vi "UiSchematic_b2g1.vi"() -> ()   [LabVIEW 2011]
uses:
  VentilS.ctl
  Pumpe.ctl
  MR.ctl
  Regelventil.ctl
  Output - Cluster b2g1.ctl
  <vilib>/Platform/TimedLoop/XDataNode/timing_clust.ctl
  <vilib>/Platform/TimedLoop/XDataNode/nitl_modes.ctl
  <vilib>/Platform/TimedLoop/XDataNode/wakeup.ctl
  <vilib>/Platform/TimedLoop/XDataNode/XDataNode.xnode
  <vilib>/Platform/TimedLoop/XDataNode/XDNodeRunTimeDep.lvlib
panel:
  out "V-13":T1
  out "V-15":T1
  out "P-9":bool
  out "target connection":bool
  out "TS-6 [°C]":dbl format="%.2g"
  out "HS-2":bool
  in  "Output Var B2G1":refnum<k21>="ni.var.psp://10.27.40.24/variables - b2g1/data - network - b2g1"
  in  "stop":bool
  out "P-4 ERR":bool
  out "P-5 ERR":bool
  out "TS-5 [°C]":dbl format="%.2g"
  out "P-4":T2
  out "DFS-1 [dl]":u64
  out "DFS-1 [l/min]":dbl format="%.2f"
  out "P-4 [%]":u8
  out "P-5 [%]":u8
  out "V-14":T3
  out "V-33":T3
  out "HS-1":bool
  out "pHS-1 [pH]":dbl format="%.2g"
  out "TS-4 [°C]":dbl format="%.2g"
  out "DS-1 [bar]":dbl format="%.2g"
  out "V-13":u8
  out "V-15":u8
  out "P-5":T2
  out "T-2 Max!":bool
  out "T-2 Min!":bool
  out "T-1 Min!":bool
  out "T-1 Max!":bool
  out "V-10":T3
  out "MR Min!":bool
  out "MR Max!":bool
  out "V-34":T3
  out "FS-1 [l]":dbl(slide) scale=10.0..80.0 scale format="%#.2g"
  out "FS-2 [l]":dbl(slide) scale=10.0..80.0 scale format="%#.2g"
  out "FS-3 [l]":T4 scale=0.0..5.0 scale format="%#.1g"
  # "B2G1"
  # "T-3"
  # "T-1"
  # "MR"
  # "T-2"
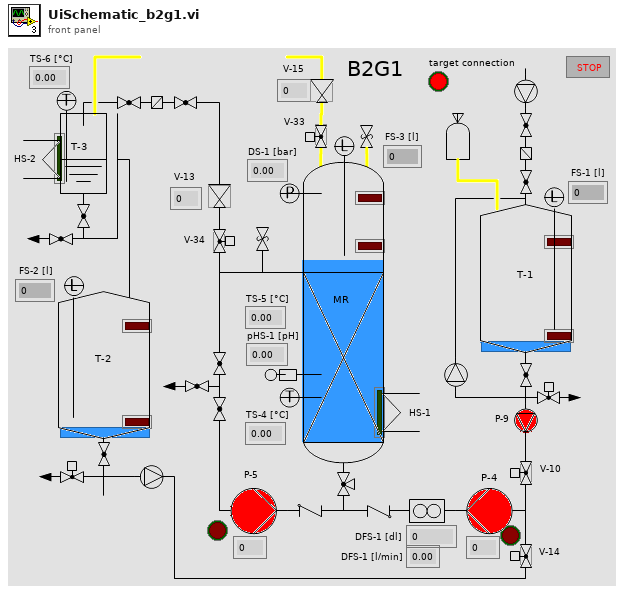
[diagram p1: front panel]
types:
  T1 = typedef "Regelventil.ctl" = bool
  T2 = typedef "Pumpe.ctl" = bool
  T3 = typedef "VentilS.ctl" = bool
  T4 = typedef "MR.ctl" = dbl
  T5 = typedef "Output - Cluster b2g1.ctl" = cluster{"DFS-1 [dl]":u64, "FS-3 [l]":dbl, "DFS-1 [l/min]":dbl, "DS-1 [bar]":dbl, "V-10 ZU":bool, "V-14 ZU":bool, "FS-1 [l]":dbl, "FS-2 [l]":dbl, "TS-4 [°C]":dbl, "HS-1":bool, "V-13 [%]":u8, "V-15 [%]":u8, "P-4 [%]":u8, "P-5 [%]":u8, "Dosierung":bool, "MR Max Füllstand":bool, "MR Min Füllstand":bool, "Dosiermenge [l]":sgl, "V-14 AUF":bool, "V-10 AUF":bool, "T-1 Max Füllstand":bool, "T-1 Min Füllstand":bool, "T-2 Max Füllstand":bool, "T-2 Min Füllstand":bool, "pHS-1 [pH]":dbl, "P-4 RUN":bool, "P-5 RUN ":bool, "V-33 AUF":bool, "V-33 ZU":bool, "V-34 AUF":bool, "V-34 ZU":bool, "P-4 ERR":bool, "P-5 ERR":bool, "TS-5 [°C]":dbl, "TS-6 [°C]":dbl, "P-9 RUN":bool, "HS-2":bool}
  T6 = typedef "XDNodeRunTimeDep.lvlib/timing_clust.ctl" = cluster{"Expected End [f-1]":u64, "Actual End [f-1]":u64, "Finished Late? [f-1]":bool, "Expected End [i-1]":u64, "Actual End [i-1]":u64, "Finished Late? [i-1]":bool, "Expected Start [i]":u64, "Actual Start [i]":u64, "Expected Start [f]":u64, "Actual Start [f]":u64, "Source Name":string, "Structure Name":string, "Period":i64, "Deadline":i64, "Offset":i64, "Start":i64, "Priority":i32, "Timeout":i32, "Mode":T7, "Wakeup Reason":T8, "Error":errorcluster, "Source Type":string, "Secondary Source Type":string, "Global End Time":u64, "Global Start Time":u64, "Frame Duration":u64, "Iteration Duration":u64, "Assigned CPU":i32, "I/O Scan Engine Mode":u32}
  T7 = typedef "XDNodeRunTimeDep.lvlib/nitl_modes.ctl" = enum32{"No Change", "Process missed periods, maintain original phase", "Discard missed periods, maintain original phase", "Process missed periods, ignore original phase", "Discard missed periods, ignore original phase"}
  T8 = typedef "XDNodeRunTimeDep.lvlib/wakeup.ctl" = enum32{"Normal", "Aborted", "Asynchronous wakeup", "Timing source error", "Timed loop error", "Timeout"}
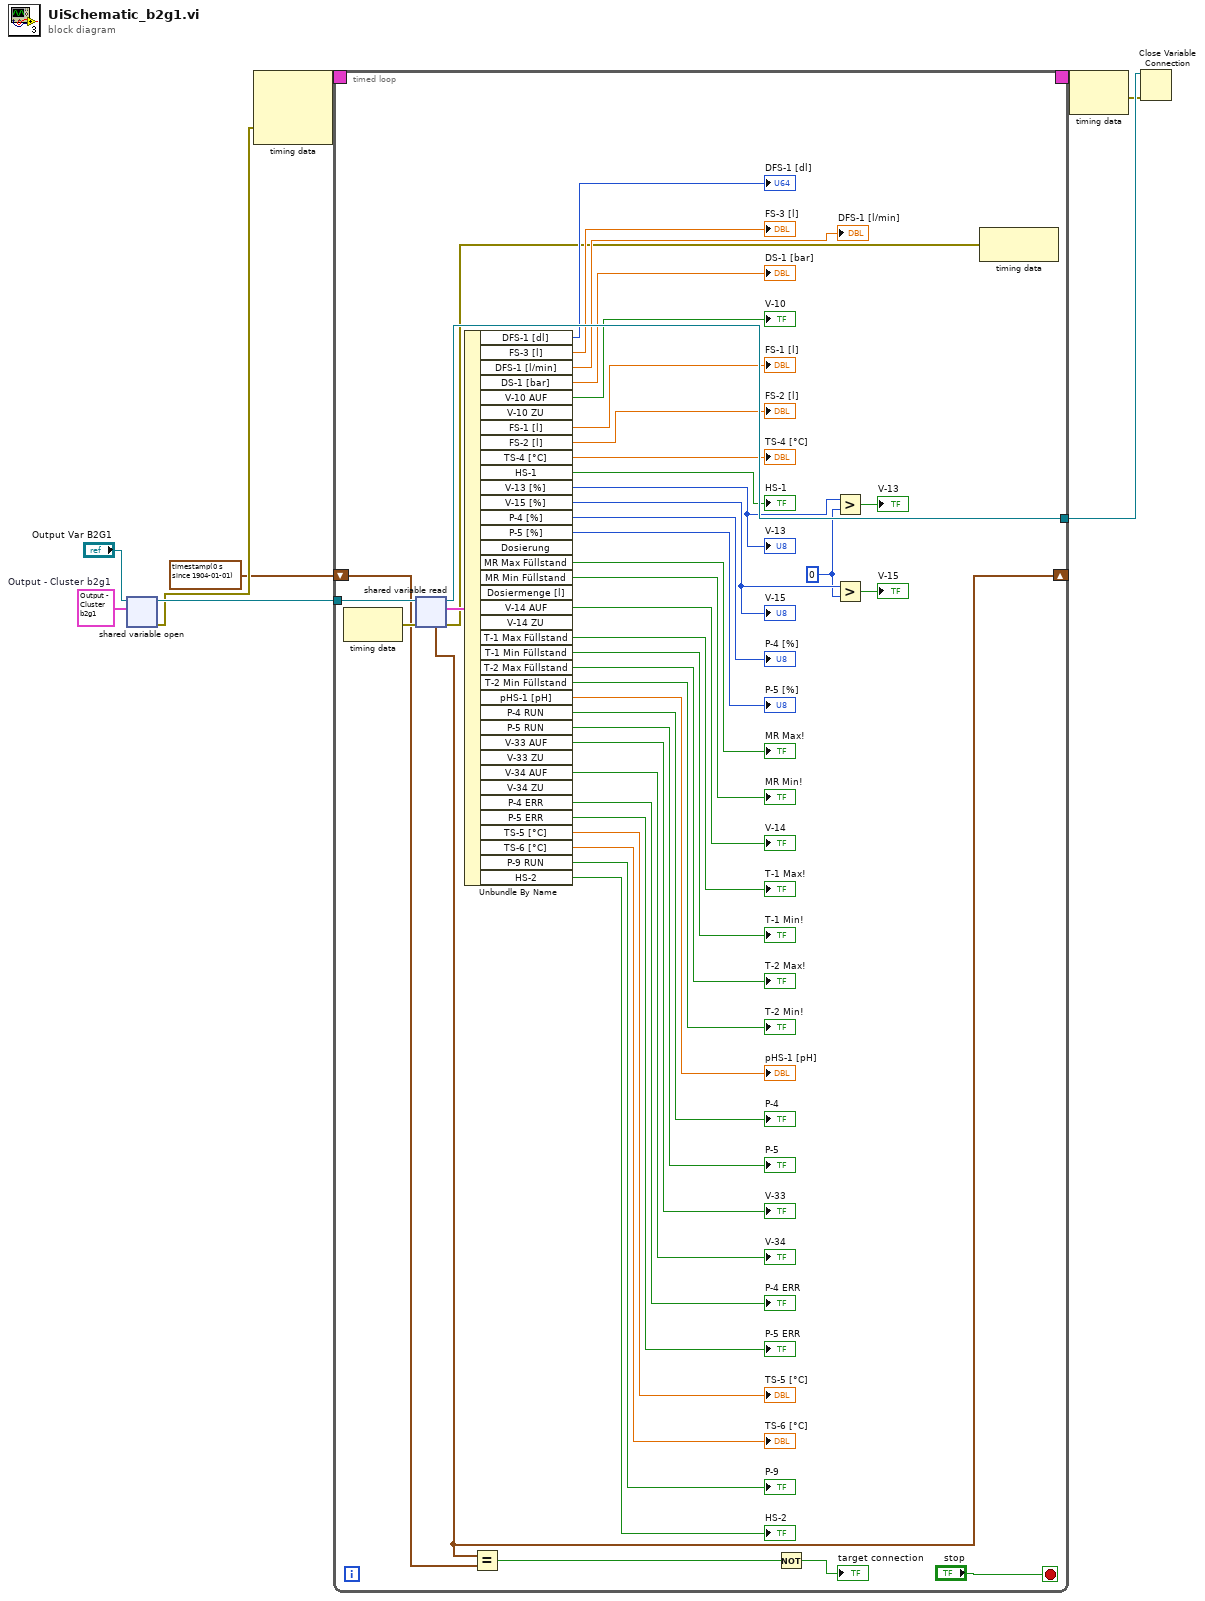
[diagram p0: block diagram]
diagram:
  w7 = T5 {"DFS-1 [dl]"=0, "FS-3 [l]"=0.0, "DFS-1 [l/min]"=0.0, "DS-1 [bar]"=0.0, "V-10 ZU"=FALSE, "V-14 ZU"=FALSE, "FS-1 [l]"=0.0, "FS-2 [l]"=0.0, "TS-4 [°C]"=0.0, "HS-1"=FALSE, "V-13 [%]"=0, "V-15 [%]"=0, "P-4 [%]"=0, "P-5 [%]"=0, "Dosierung"=FALSE, "MR Max Füllstand"=FALSE, "MR Min Füllstand"=FALSE, "Dosiermenge [l]"=0.0, "V-14 AUF"=FALSE, "V-10 AUF"=FALSE, "T-1 Max Füllstand"=FALSE, "T-1 Min Füllstand"=FALSE, "T-2 Max Füllstand"=FALSE, "T-2 Min Füllstand"=FALSE, "pHS-1 [pH]"=0.0, "P-4 RUN"=FALSE, "P-5 RUN "=FALSE, "V-33 AUF"=FALSE, "V-33 ZU"=FALSE, "V-34 AUF"=FALSE, "V-34 ZU"=FALSE, "P-4 ERR"=FALSE, "P-5 ERR"=FALSE, "TS-5 [°C]"=0.0, "TS-6 [°C]"=0.0, "P-9 RUN"=FALSE, "HS-2"=FALSE}  # Output - Cluster b2g1
  n1 = shared-variable-open("Output Var B2G1", w7) -> (w8:refnum<k21>, w2:errorcluster)  [unwired: 2 in]
  n2 = node-c288(w2) -> (w5:T6)  [unwired: 2 in]
  n3 = timed-loop {
    timing: w5 -> [_]
    timing-out: [_] -> w4
    tunnel: w8 -> [w53]
    tunnel: [w52] -> w6
    shift-right: [w21] -> _
    shift-left: timestamp(0 s since 1904-01-01) -> [w22]
    stop <- "stop" stop-if-true
    w31 = u8 0 ("y")
    n4 = node-c288() -> (w28:errorcluster)  [unwired: 1 in]
    n5 = shared-variable-read(w53, w28) -> (w52:refnum<k21>, w27:errorcluster, w29:T5, w21:timestamp)
    n6 = Unbundle By Name(w29) -> ("DFS-1 [dl]"=→"DFS-1 [dl]":u64, "FS-3 [l]"=→"FS-3 [l]":dbl, "DFS-1 [l/min]"=→"DFS-1 [l/min]":dbl, "DS-1 [bar]"=→"DS-1 [bar]":dbl, "V-10 AUF"=→"V-10":bool, "FS-1 [l]"=→"FS-1 [l]":dbl, "FS-2 [l]"=→"FS-2 [l]":dbl, "TS-4 [°C]"=→"TS-4 [°C]":dbl, "HS-1"=→"HS-1":bool, "V-13 [%]"=w30:u8, "V-15 [%]"=w32:u8, "P-4 [%]"=→"P-4 [%]":u8, "P-5 [%]"=→"P-5 [%]":u8, "MR Max Füllstand"=→"MR Max!":bool, "MR Min Füllstand"=→"MR Min!":bool, "V-14 AUF"=→"V-14":bool, "T-1 Max Füllstand"=→"T-1 Max!":bool, "T-1 Min Füllstand"=→"T-1 Min!":bool, "T-2 Max Füllstand"=→"T-2 Max!":bool, "T-2 Min Füllstand"=→"T-2 Min!":bool, "pHS-1 [pH]"=→"pHS-1 [pH]":dbl, "P-4 RUN"=→"P-4":bool, "P-5 RUN"=→"P-5":bool, "V-33 AUF"=→"V-33":bool, "V-34 AUF"=→"V-34":bool, "P-4 ERR"=→"P-4 ERR":bool, "P-5 ERR"=→"P-5 ERR":bool, "TS-5 [°C]"=→"TS-5 [°C]":dbl, "TS-6 [°C]"=→"TS-6 [°C]":dbl, "P-9 RUN"=→"P-9":bool, "HS-2"=→"HS-2":bool)  [unwired: 6 out]
    "V-15" <- w32
    "V-13" <- w30
    n7 = Equal?(x=w21, y=w22) -> (x = y?=w19:bool)
    n8 = Not(x=w19) -> (.not. x?=→"target connection":bool)
    n9 = Greater?(x=w30, y=w31) -> (0:→"V-13":bool)
    n10 = Greater?(x=w32, y=w31) -> (0:→"V-15":bool)
    n11 = node-c288(w27) -> ()  [unwired: 1 out]
  }
  n12 = node-c288(w4) -> (w3:errorcluster)
  n13 = Close Variable Connection(8:w3, 11:w6) -> ()  [unwired: 1 out]
